vi "UDP Tx Process.vi"(10 "Parameters":variant, 11 "Process":refnum<class "Process.lvclass">) -> ()   [LabVIEW 2016, in "UDP-Custom-Device Engine.lvlib"]
uses:
  UDP-Custom-Device Engine.lvlib
  <vilib>/NI/NIVS Inline Async API/_VS Inline Async API/Process/Process.lvclass
  <vilib>/NI/NIVS Inline Async API/_VS Inline Async API/Process/Process.lvclass/Process.ctl
  <vilib>/NI/NIVS Inline Async API/_Data Access Engine/Access Type Classes/Read/Read.lvclass/Read.ctl
  <vilib>/NI/NIVS Inline Async API/_Data Access Engine/Data Access Engine/Methods/Read.Data.vi
  <vilib>/NI/NIVS Inline Async API/_VS Inline Async API/Process/Data Member Access/Read Data Access.vi
  <vilib>/NI/NIVS Inline Async API/_VS Inline Async API/Error Handling Process/SubVIs/Error.ConvertArray.vi
  <vilib>/NI/NIVS Inline Async API/_Data Access Engine/Access Type Classes/Read/Read.ProcessData.vi
  <vilib>/NI/NIVS Inline Async API/_Data Access Engine/Data Access Engine/Data Access Engine.lvclass
  <vilib>/NI/NIVS Inline Async API/_Data Access Engine/Access Type Classes/Read/Read.lvclass
  <vilib>/NI Veristand/VeriStand Data/Library/Byte Buffer/Byte Buffer.lvclass
  <vilib>/NI/NIVS Inline Async API/_Data Access Engine/Access Type Classes/ReadWrite/ReadWrite.lvclass
  <vilib>/NI Veristand/VeriStand Data/Library/VeriStand Data.lvlib
panel:
  out "length":i32
  out "Tx Packet":string
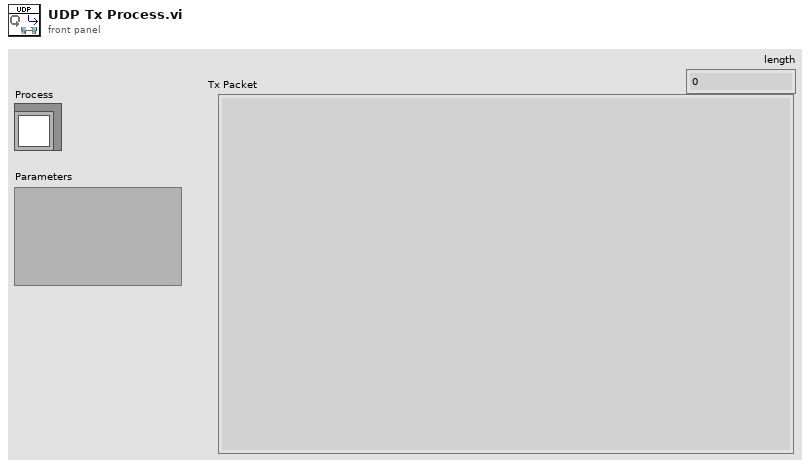
[diagram p1: front panel]
types:
  T1 = typedef "UDP-Custom-Device Engine.lvlib/Engine - Tx Loop Data.ctl" = cluster{"Packet Name":string, "Packet ID":i32, "Loop Period":u32, "Destination IP Address":u32, "Destination Port":u16, "Tx FIFO Ref":T2, "Connection ID":refnum<k16>, "Local IP Address":string, "Local Port":i32, "Byte Order":enum16{"big-endian, network order", "native, host order", "little-endian"}, "Always Transmit":bool, "TTL":u16, "Multicast":bool, "Multicast IP Address":u32, "Header Info":bool[], "Channel Data Types":T3[], "Data Conversion":T4, "Header Details":T6, "Transmit Ref":T7}
  T2 = typedef "Data Access Engine.lvlib/Data Access Engine.lvclass/Read.DVR.ctl" = refnum<data-value>
  T3 = typedef "VeriStand Data.lvlib/Typedefs.Data Types.ctl" = enum16{"Boolean", "Single", "Double", "I8", "I16", "I32", "I64", "U8", "U16", "U32", "U64"}
  T4 = typedef "UDP-Custom-Device Engine.lvlib/Engine - Data Conversion Config.ctl" = cluster{"Byte Buffer":refnum<class "Byte Buffer.lvclass">, "Data Pointers":u64[], "Channel Count":i32, "Mappings":T5[], "Static Header Payload":string, "Packet Count":dbl, "Packet Size":i32}
  T5 = typedef "VeriStand Data.lvlib/Byte Buffer.lvclass/Byte Buffer.Mapping.ctl" = cluster{"pointer":u64, "count":i32, "buffer offset":i32, "data type":T3}
  T6 = typedef "UDP-Custom-Device Shared.lvlib/Shared - Header Details.ctl" = cluster{"Packet Size":u16, "Protocol Revision":u8, "System Definition Version":u64, "Source Node Name":string, "Packet ID":u32, "Number of Channels":u32, "Static Header Size":u16, "Total Header Size":u16}
  T7 = typedef "Data Access Engine.lvlib/Data Access Engine.lvclass/ReadWrite.DVR.ctl" = refnum<data-value>
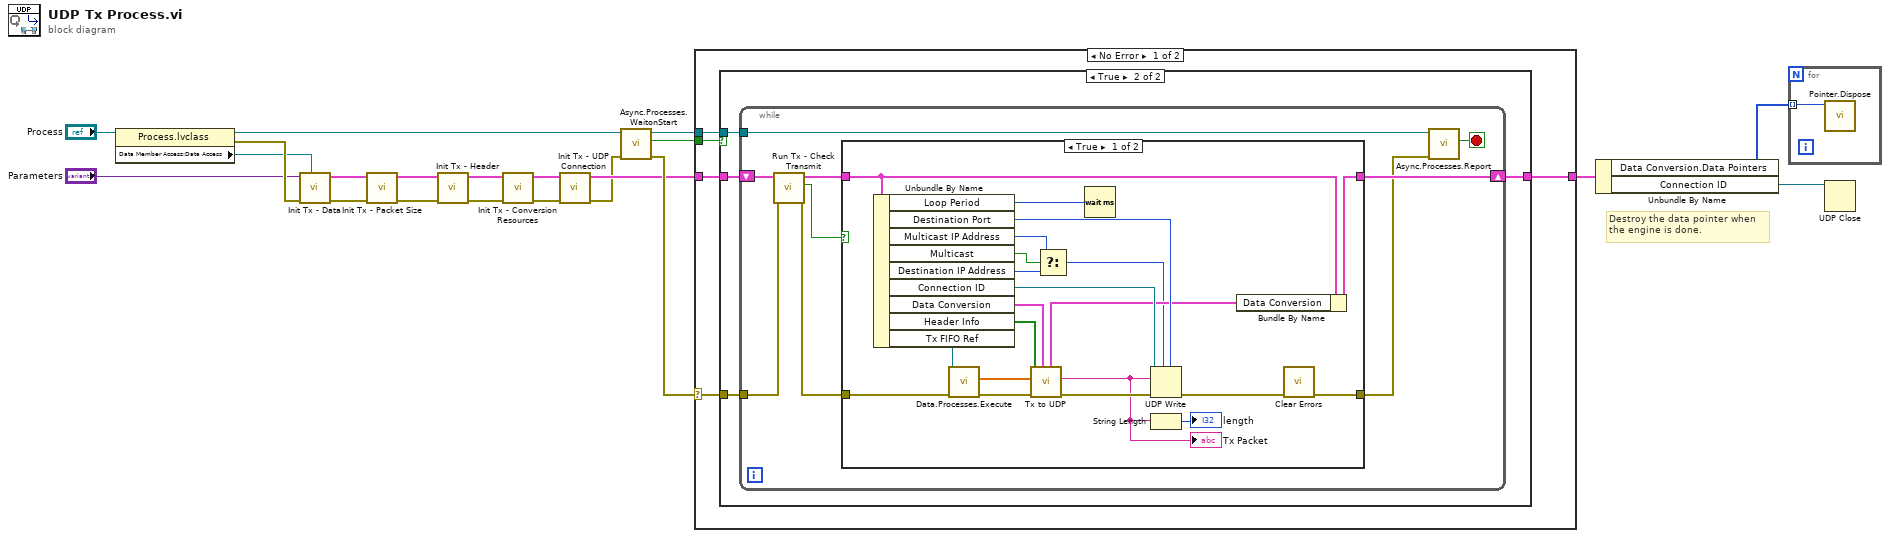
[diagram p0: block diagram]
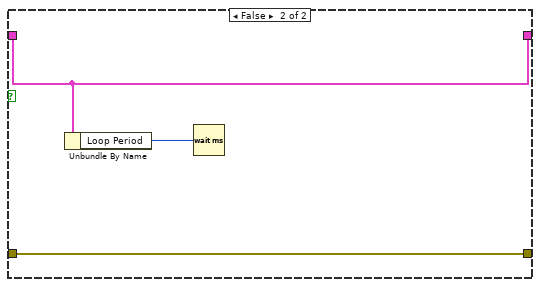
[diagram p3: hidden frame]
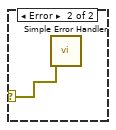
[diagram p4: hidden frame]
diagram:
  # "Destroy the data pointer when\nthe engine is done."
  n1 = property class="Process.lvclass"(reference="Process") -> (reference out=w21:refnum<class "Process.lvclass">, error out=w16:errorcluster, "Data Member Access:Data Access"=w12:refnum<class "Data Access Engine.lvclass">)  [unwired: 1 in]
  n2 = call "Init Tx - Data.vi"("Data Access in"=w12, "error in (no error)"=w16, "Parameters"="Parameters") -> ("error out"=w4:errorcluster, "Tx Loop Data"=w1:T1)  [unwired: 6 in, 1 out]
  n3 = call "Init Tx - Packet Size.vi"("error in (no error)"=w4, "Tx Loop Data"=w1) -> ("error out"=w3:errorcluster, "Tx Loop Data out"=w5:T1)  [unwired: 8 in]
  n4 = call "Init Tx - Header.vi"("error in (no error)"=w3, "Tx Loop Data"=w5) -> ("error out"=w6:errorcluster, "Tx Loop Data out"=w7:T1)  [unwired: 8 in]
  n5 = call "Init Tx - Conversion Resources.vi"("error in (no error)"=w6, "Tx Loop Data"=w7) -> ("error out"=w10:errorcluster, "Tx Loop Data out"=w11:T1)  [unwired: 8 in]
  n6 = call "Init Tx - UDP Connection.vi"("error in (no error)"=w10, "Tx Loop Data in"=w11) -> ("error out"=w13:errorcluster, "Tx Loop Data out"=w14:T1)  [unwired: 8 in]
  n7 = call <vilib>:"Async.Processes.WaitonStart.vi"("error in (no error)"=w13, "Process"=w21) -> ("error out"=w19:errorcluster, "Execute"=w17:bool, "Process out"=w18:refnum<class "Process.lvclass">)  [unwired: 7 in]
  n8 = case shown="No Error" w19 {
    selector: w19 -> [w24 w65]
    tunnel: w17 -> [w26 _]
    tunnel: w18 -> [w25 _]
    tunnel: w14 -> [w23 _]
    tunnel: [w22 _] -> w8
    frame No Error {
      n9 = case shown="True" w26 {
        tunnel: w24 -> [_ w30]
        tunnel: w25 -> [_ w31]
        tunnel: w23 -> [w27 w29]
        tunnel: [w27 w28] -> w22
        frame False {
        }
        frame True {
          n10 = while {
            tunnel: w30 -> [w35]
            tunnel: w31 -> [w40]
            shift-right: [w38] -> w28
            shift-left: w29 -> [w37]
            stop <- w39 stop-if-true
            n11 = call "Run Tx - Check Transmit.vi"("error in (no error)"=w35, "Tx Loop Data in"=w37) -> ("error out"=w34:errorcluster, "Transmit?"=w33:bool, "Tx Loop Data out"=w36:T1)  [unwired: 7 in]
            n12 = case shown="True" w33 {
              tunnel: [w45 w62] -> w32
              tunnel: [w61 w63] -> w38
              tunnel: w36 -> [w48 w63]
              tunnel: w34 -> [w47 w62]
              frame True {
                n13 = Unbundle By Name(w48) -> ("Loop Period"=w55:u32, "Destination Port"=w54:u16, "Multicast IP Address"=w42:u32, "Multicast"=w43:bool, "Destination IP Address"=w44:u32, "Connection ID"=w57:refnum<k16>, "Data Conversion"=w52:T4, "Header Info"=w53:bool[], "Tx FIFO Ref"=w56:T2)
                n14 = call-poly <vilib>:"Data.Processes.Execute.vi"("error in (no error)"=w47, "Ref"=w56) -> ("error out"=w60:errorcluster, "Values"=w59:dbl[])  [unwired: 7 in, 1 out]
                n15 = call "Tx to UDP.vi"("Data Conversion"=w52, "error in (no error)"=w60, "Tx Array"=w59, "Header Info"=w53) -> ("error out"=w58:errorcluster, "Tx String"=w50:string, "Data Conversion out"=w51:T4)  [unwired: 5 in]
                "Tx Packet" <- w50
                n16 = Select(t=w42, s=w43, f=w44) -> (s? t:f=w41:u32)
                n17 = Wait (ms)(milliseconds to wait=w55) -> ()  [unwired: 1 out]
                n18 = UDP Write(address=w41, port or service name=w54, connection ID=w57, data in=w50, 8:w58) -> (error out=w46:errorcluster)  [unwired: 1 in, 1 out]
                n19 = String Length(string=w50) -> (length=→"length":i32)
                n20 = Bundle By Name(cluster=w48, "Data Conversion"=w51) -> (w61:T1)
                n21 = call <vilib>:"Clear Errors.vi"("error in (no error)"=w46) -> ("error out"=w45:errorcluster)  [unwired: 5 in, 1 out]
              }
              frame False {
                n22 = Unbundle By Name(w63) -> ("Loop Period"=w64:u32)
                n23 = Wait (ms)(milliseconds to wait=w64) -> ()  [unwired: 1 out]
              }
            }
            n24 = call <vilib>:"Async.Processes.Report.vi"("Error"=w32, "Process in"=w40) -> ("Stop"=w39:bool)  [unwired: 8 in, 1 out]
          }
        }
      }
    }
    frame Error {
      n25 = call <vilib>:"Simple Error Handler.vi"("error in (no error)"=w65) -> ()  [unwired: 4 in, 5 out]
    }
  }
  n26 = Unbundle By Name(w8) -> ("Data Conversion.Data Pointers"=w9:u64[], "Connection ID"=w2:refnum<k16>)
  n27 = for {
    tunnel: w9 -> [w66] mode=indexing
    n28 = call <vilib>:"Pointer.Dispose.vi"("pointer"=w66) -> ()  [unwired: 9 in, 2 out]
  }
  n29 = UDP Close(connection ID=w2) -> ()  [unwired: 1 in, 2 out]
